vi "Add Leaf to Branch.vi"(8 "error in":errorcluster, 9 "Item":variant, 10 "Name":string, 11 "Tree in":refnum<class "Tree.lvclass">) -> (0 "error out":errorcluster, 3 "Tree out":refnum<class "Tree.lvclass">)   [LabVIEW 2019, in "Tree.lvclass"]
uses:
  Tree.lvclass
  Tree.lvclass/Tree.ctl
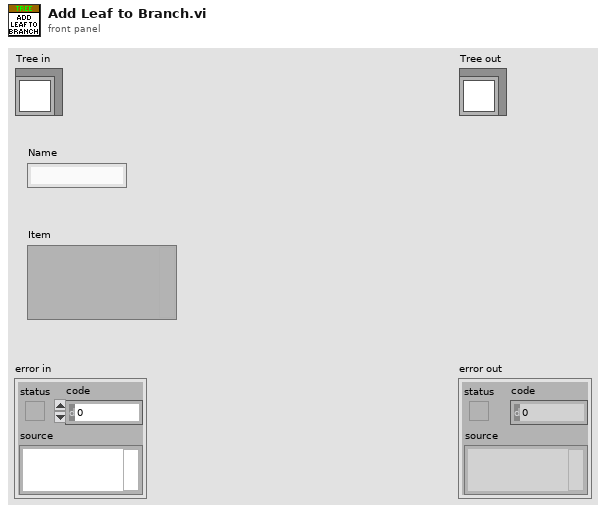
[diagram p1: front panel]
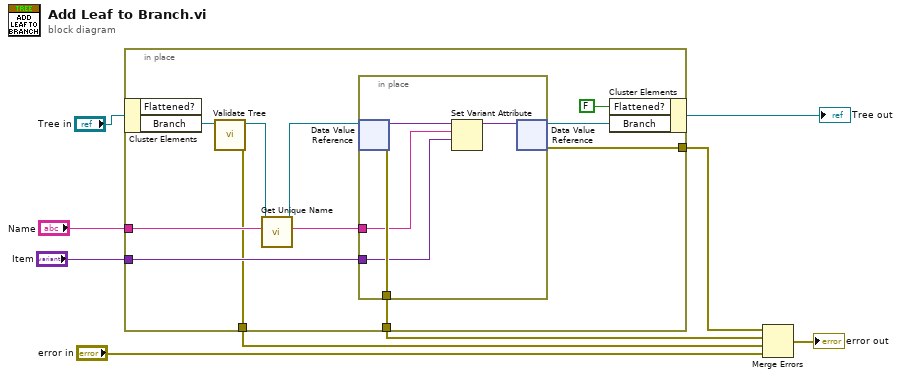
[diagram p0: block diagram]
diagram:
  n1 = in-place {
    in-place-border: [w19] -> w5
    in-place-border: [w10] -> w3
    in-place-border: [w18] -> w4
    in-place-border: "Name" -> [w16]
    in-place-border: "Item" -> [w14]
    n2 = in-place-cluster #1("Tree in") -> ("Branch"=w12:refnum<data-value>)  [unwired: 1 out]
    n3 = call "Validate Tree.vi"("Branch Reference In"=w12) -> ("error out"=w10:errorcluster, "Branch Reference Out"=w11:refnum<data-value>)  [unwired: 9 in]
    n4 = call "Get Unique Name.vi"("Name"=w16, "Branch"=w11) -> ("Unique Name"=w15:string, "Branch"=w17:refnum<data-value>)  [unwired: 7 in, 1 out]
    n5 = in-place {
      in-place-border: [w25] -> w18
      in-place-border: w15 -> [w22]
      in-place-border: w14 -> [w21]
      n6 = in-place-dvr #2(w17) -> (w24:variant, w25:errorcluster)
      n7 = Set Variant Attribute(Variant=w24, name=w22, value=w21) -> (Variant out=w23:variant)  [unwired: 1 in, 2 out]
      n8 = in-place-dvr #2(w23) -> (w20:refnum<data-value>, w19:errorcluster)
    }
    n9 = in-place-cluster #1("Flattened?"=FALSE ("Flattened Up to Date?"), "Branch"=w20) -> (→"Tree out":refnum<class "Tree.lvclass">)
  }
  n10 = Merge Errors(w5, w4, w3, "error in") -> (→"error out":errorcluster)
